vi "AlliGator Read metadata.txt File.vi"(8 "Error In":errorcluster, 11 "Folder Path":path) -> (0 "Error Out":errorcluster, 1 "Metadata":T1 {"Date" format="%<%x %.3X>T"}, 2 "AlliGator Version":string, 3 "Settings String":string)   [LabVIEW 2021, in "AlliGator Files.lvlib"]
doc: "Tries to extract FLI dataset metadata from a _metadata.txt file generated by AlliGator."
uses:
  AlliGator Files.lvlib
  AlliGator RecSettings Metadata.ctl
  AlliGator Gate Folder Metadata List.ctl
panel:
  # "see the AlliGator License on the block diagram (Ctrl+E or Window:Show Block Diagram)"
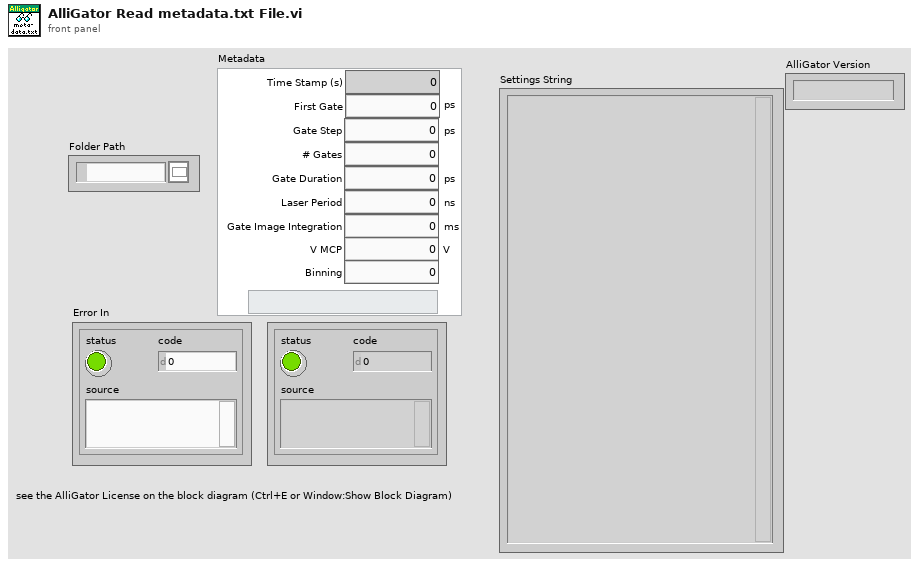
[diagram p1: front panel]
types:
  T1 = typedef "AlliGator Files.lvlib/AlliGator RecSettings Metadata.ctl" = cluster{"Time Stamp (s)":dbl, "First Gate":dbl[unit], "Gate Step":dbl[unit], "# Gates":i32, "Gate Duration":dbl[unit], "Laser Period":dbl[unit], "Gate Image Integration":dbl[unit], "Date":timestamp, "V MCP":dbl[unit], "Binning":dbl}
  T2 = typedef "AlliGator Files.lvlib/AlliGator Gate Folder Metadata List.ctl" = enum16{"[DAQ Parameters]", "DAQ Parameters.# Pixel X", "DAQ Parameters.# Pixel Y", "DAQ Parameters.# Gates", "DAQ Parameters.# Datasets", "DAQ Parameters.Exposure/Gate", "DAQ Parameters.Macrotime Gate Separation", "DAQ Parameters.Nanotime Gate Separation", "DAQ Parameters.Gate Duration", "DAQ Parameters.Laser Period", "[Dataset Timestamp]", "Timestamp", "[Metadata]", "AlliGator Version"}
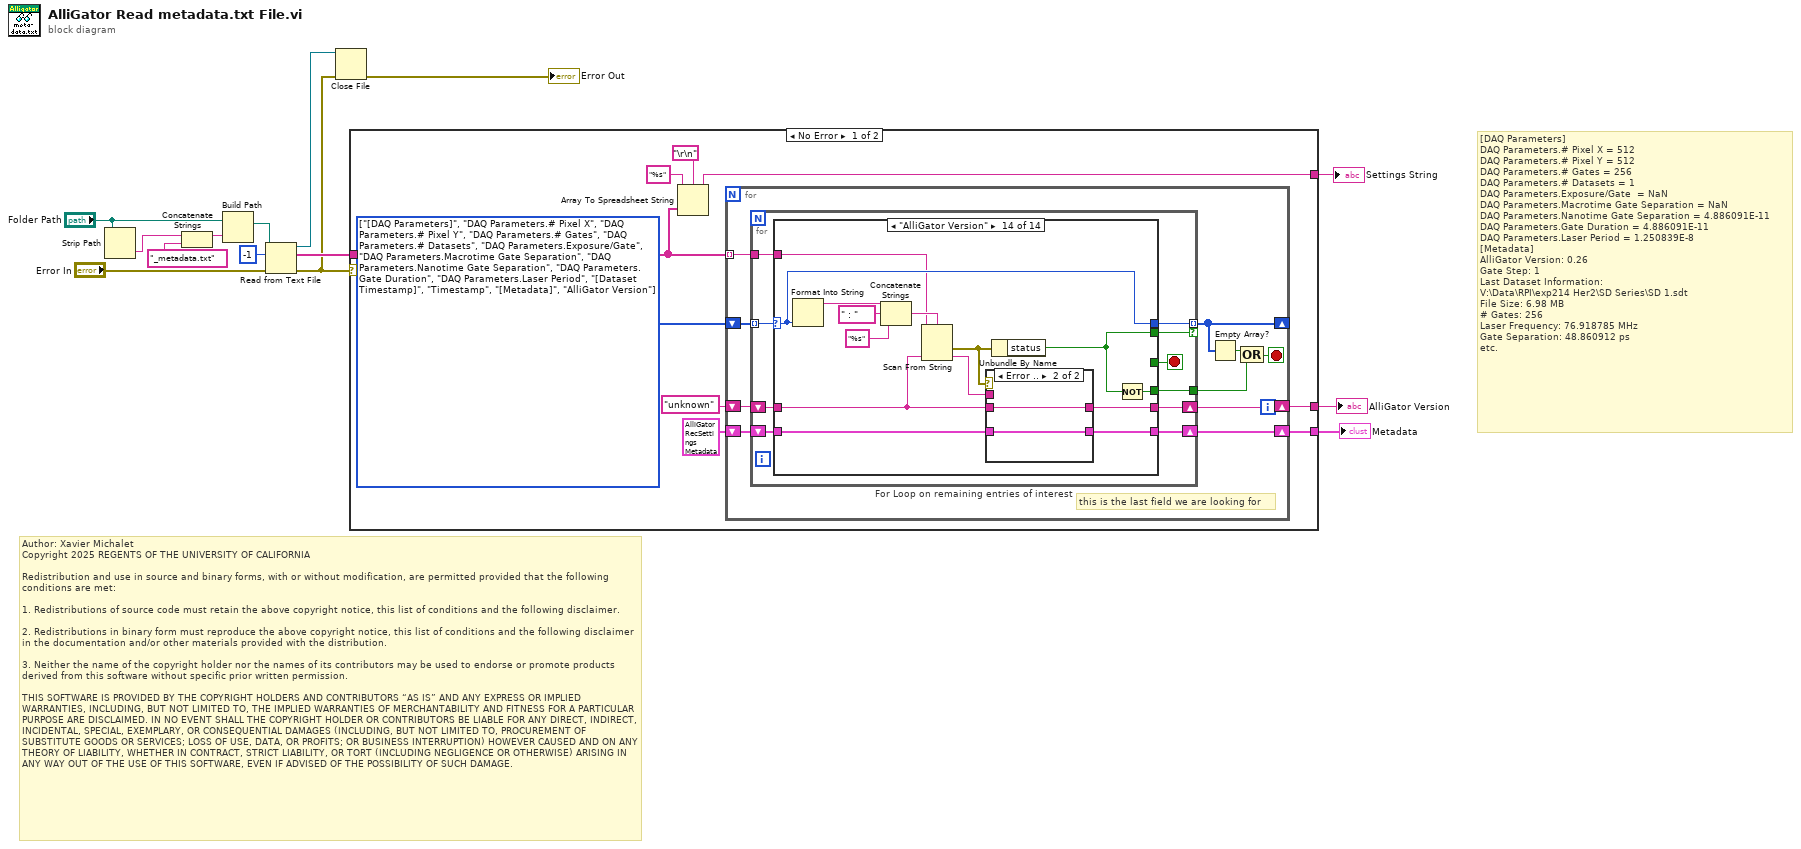
[diagram p0: block diagram]
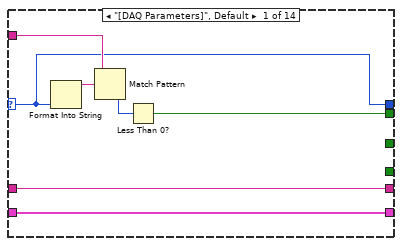
[diagram p2: hidden frame]
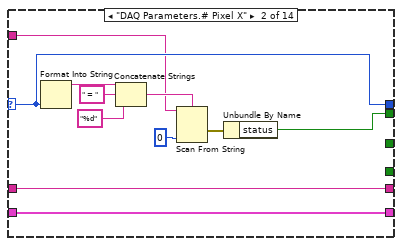
[diagram p3: hidden frame]
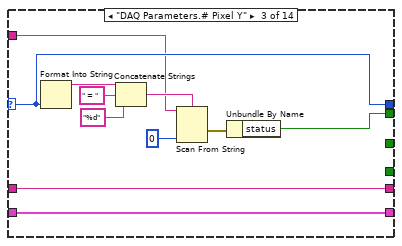
[diagram p4: hidden frame]
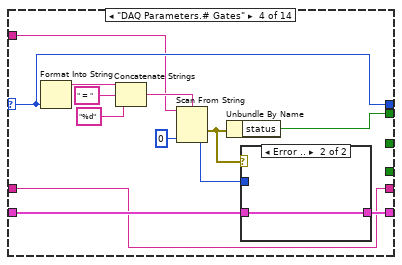
[diagram p5: hidden frame]
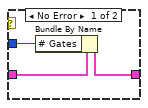
[diagram p6: hidden frame]
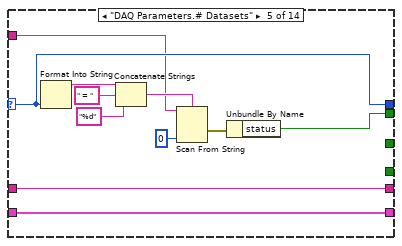
[diagram p7: hidden frame]
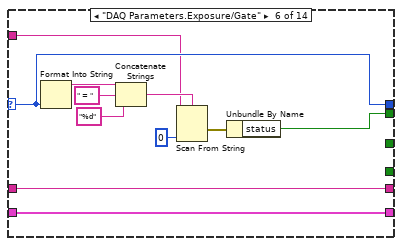
[diagram p8: hidden frame]
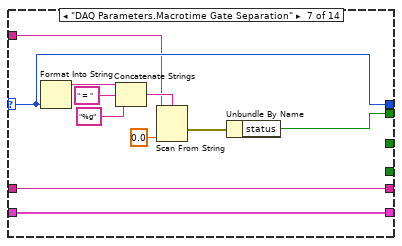
[diagram p9: hidden frame]
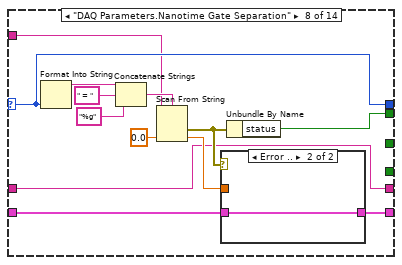
[diagram p10: hidden frame]
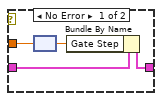
[diagram p11: hidden frame]
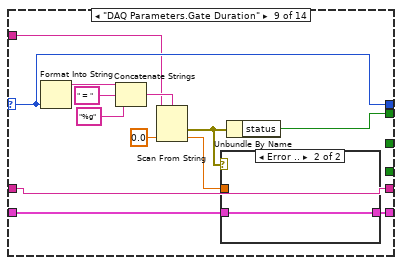
[diagram p12: hidden frame]
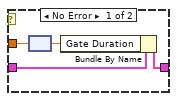
[diagram p13: hidden frame]
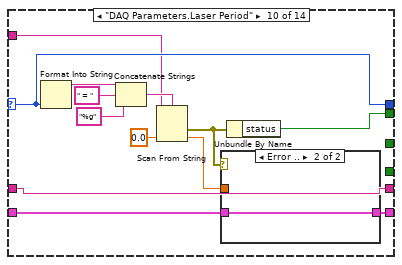
[diagram p14: hidden frame]
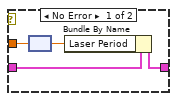
[diagram p15: hidden frame]
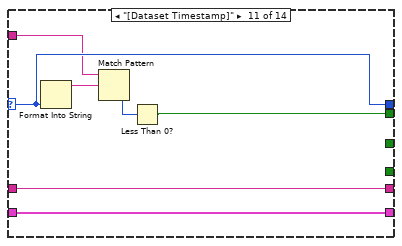
[diagram p16: hidden frame]
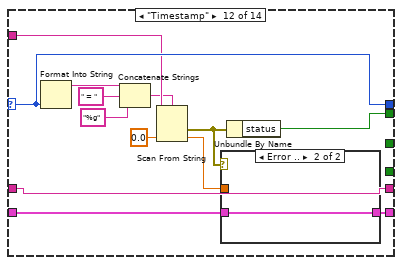
[diagram p17: hidden frame]
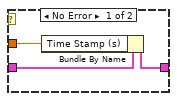
[diagram p18: hidden frame]
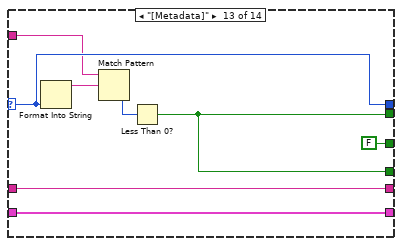
[diagram p19: hidden frame]
diagram:
  # "Author: Xavier Michalet\nCopyright 2025 REGENTS OF THE UNIVERSITY OF CALIFORNIA\n\nRedistribution and use in source and binary forms, with or without modification, are permitted provided that the following conditions are met:\n\n1. Redistributions of source code must retain the above copyright notice, this list of conditions and the following disclaimer.\n\n2. Redistributions in binary form must reproduce the above copyright notice, this list of conditions and the following disclaimer in the documentation and/or other materials provided with the distribution.\n\n3. Neither the name of the copyright holder nor the names of its contributors may be used to endorse or promote products derived from this software without specific prior written permission.\n\nTHIS SOFTWARE IS PROVIDED BY THE COPYRIGHT HOLDERS AND CONTRIBUTORS “AS IS” AND ANY EXPRESS OR IMPLIED WARRANTIES, INCLUDING, BUT NOT LIMITED TO, THE IMPLIED WARRANTIES OF MERCHANTABILITY AND FITNESS FOR A PARTICULAR PURPOSE ARE DISCLAIMED. IN NO EVENT SHALL THE COPYRIGHT HOLDER OR CONTRIBUTORS BE LIABLE FOR ANY DIRECT, INDIRECT, INCIDENTAL, SPECIAL, EXEMPLARY, OR CONSEQUENTIAL DAMAGES (INCLUDING, BUT NOT LIMITED TO, PROCUREMENT OF SUBSTITUTE GOODS OR SERVICES; LOSS OF USE, DATA, OR PROFITS; OR BUSINESS INTERRUPTION) HOWEVER CAUSED AND ON ANY THEORY OF LIABILITY, WHETHER IN CONTRACT, STRICT LIABILITY, OR TORT (INCLUDING NEGLIGENCE OR OTHERWISE) ARISING IN ANY WAY OUT OF THE USE OF THIS SOFTWARE, EVEN IF ADVISED OF THE POSSIBILITY OF SUCH DAMAGE."
  # "[DAQ Parameters]\nDAQ Parameters.# Pixel X = 512\nDAQ Parameters.# Pixel Y = 512\nDAQ Parameters.# Gates = 256\nDAQ Parameters.# Datasets = 1\nDAQ Parameters.Exposure/Gate  = NaN\nDAQ Parameters.Macrotime Gate Separation = NaN\nDAQ Parameters.Nanotime Gate Separation = 4.886091E-11\nDAQ Parameters.Gate Duration = 4.886091E-11\nDAQ Parameters.Laser Period = 1.250839E-8\n[Metadata]\nAlliGator Version: 0.26\nGate Step: 1\nLast Dataset Information:\nV:\\Data\\RPI\\exp214 Her2\\SD Series\\SD 1.sdt\nFile Size: 6.98 MB\n# Gates: 256\nLaser Frequency: 76.918785 MHz\nGate Separation: 48.860912 ps\netc."
  n1 = Strip Path(path="Folder Path") -> (name=w4:string)  [unwired: 1 out]
  n2 = Concatenate Strings(w4, "_metadata.txt" ("name or relative path")) -> (w2:string)
  n3 = Build Path(base path="Folder Path", name or relative path=w2) -> (appended path=w10:path)
  n4 = Read from Text File(file (use dialog)=w10, count=-1, error in="Error In") -> (refnum out=w14:refnum<file>, text=w13:string[], error out=w8:errorcluster)  [unwired: 1 in, 1 out]
  n5 = Close File(refnum=w14, error in=w8) -> (error out=→"Error Out":errorcluster)  [unwired: 1 out]
  n6 = case shown="No Error" w8 {
    tunnel: w13 -> [w20 _]
    tunnel: [w22 "No metadata  found..." ("spreadsheet string")] -> w12
    tunnel: [w18 _] -> w7
    tunnel: [w16 "unknown" ("string")] -> w1
    frame No Error {
      w19 = T2[] [enum."[DAQ Parameters]", enum."DAQ Parameters.# Pixel X", enum."DAQ Parameters.# Pixel Y", enum."DAQ Parameters.# Gates", enum."DAQ Parameters.# Datasets", enum."DAQ Parameters.Exposure/Gate", enum."DAQ Parameters.Macrotime Gate Separation", enum."DAQ Parameters.Nanotime Gate Separation", enum."DAQ Parameters.Gate Duration", enum."DAQ Parameters.Laser Period", enum."[Dataset Timestamp]", enum."Timestamp", enum."[Metadata]", enum."AlliGator Version"] items=["[DAQ Parameters]", "DAQ Parameters.# Pixel X", "DAQ Parameters.# Pixel Y", "DAQ Parameters.# Gates", "DAQ Parameters.# Datasets", "DAQ Parameters.Exposure/Gate", "DAQ Parameters.Macrotime Gate Separation", "DAQ Parameters.Nanotime Gate Separation", "DAQ Parameters.Gate Duration", "DAQ Parameters.Laser Period", "[Dataset Timestamp]", "Timestamp", "[Metadata]", "AlliGator Version"] ("Array")
      n7 = Array To Spreadsheet String(delimiter (Tab)="\r\n", array=w20, 3:"%s" ("format string")) -> (spreadsheet string=w22:string)
      n8 = for {
        shift-right: [w31] -> w18
        shift-left: T1 {"Time Stamp (s)"=nan, "First Gate"=nan, "Gate Step"=nan, "# Gates"=0, "Gate Duration"=nan, "Laser Period"=nan, "Gate Image Integration"=nan, "Date"=timestamp(0 s since 1904-01-01), "V MCP"=nan, "Binning"=nan} ("Metadata") -> [w32]
        tunnel: w20 -> [w30] mode=indexing
        shift-right: [w29] -> _
        shift-left: w19 -> [w33]
        shift-right: [w24] -> w16
        shift-left: "unknown" ("string") -> [w25]
        stop <- w27 stop-if-true
        # "this is the last field we are looking for"
        n9 = for "For Loop on remaining entries of interest" {
          tunnel: w33 -> [w43] mode=indexing
          shift-right: [w41] -> w31
          shift-left: w32 -> [w42]
          tunnel: w30 -> [w40]
          tunnel: [w39] -> w29 mode=indexing if=w37
          tunnel: [w36] -> w26
          shift-right: [w34] -> w24
          shift-left: w25 -> [w35]
          stop <- w38 stop-if-true
          n10 = case shown="\"AlliGator Version\"" w43 {
            selector: w43 -> [w47 w61 w72 w85 w100 w111 w122 w135 w153 w171 w183 w196 w208 w222]
            tunnel: w42 -> [w45 w60 w71 w77 w92 w103 w113 w126 w144 w162 w182 w191 w207 w215]
            tunnel: [w45 w60 w71 w76 w92 w103 w113 w125 w143 w161 w182 w190 w207 w214] -> w41
            tunnel: w40 -> [w49 w55 w66 w80 w95 w106 w117 w130 w148 w166 w179 w195 w204 w217]
            tunnel: [w47 w61 w72 w85 w100 w111 w122 w135 w153 w171 w183 w196 w208 w222] -> w39
            tunnel: [w48 w52 w63 w78 w93 w104 w115 w128 w146 w164 w178 w193 w203 w210] -> w37
            tunnel: [_ _ _ _ _ _ _ _ _ _ _ _ FALSE _] -> w38
            tunnel: [_ _ _ _ _ _ _ _ _ _ _ _ w203 w209] -> w36
            tunnel: w35 -> [w44 w51 w62 w73 w90 w101 w112 w123 w141 w159 w177 w184 w201 w211]
            tunnel: [w44 w51 w62 w73 w90 w101 w112 w123 w141 w159 w177 w184 w201 w212] -> w34
            frame "[DAQ Parameters]", Default {
              n11 = Format Into String(w47) -> (resulting string=w46:string)  [unwired: 3 in, 1 out]
              n12 = Match Pattern(string=w49, regular expression=w46) -> (offset past match=w50:i32)  [unwired: 1 in, 3 out]
              n13 = Less Than 0?(x=w50) -> (x < 0?=w48:bool)
            }
            frame "DAQ Parameters.# Pixel X" {
              n14 = Format Into String(w61) -> (resulting string=w59:string)  [unwired: 3 in, 1 out]
              n15 = Concatenate Strings(w59, " = " ("string"), "%d" ("string")) -> (w56:string)
              n16 = Scan From String(format string=w56, input string=w55, default 1=0 ("default value 1")) -> (error out=w53:errorcluster)  [unwired: 3 in, 2 out]
              n17 = Unbundle By Name(w53) -> ("status"=w52:bool)
            }
            frame "DAQ Parameters.# Pixel Y" {
              n18 = Format Into String(w72) -> (resulting string=w70:string)  [unwired: 3 in, 1 out]
              n19 = Concatenate Strings(w70, " = " ("string"), "%d" ("string")) -> (w67:string)
              n20 = Scan From String(format string=w67, input string=w66, default 1=0 ("default value 1")) -> (error out=w64:errorcluster)  [unwired: 3 in, 2 out]
              n21 = Unbundle By Name(w64) -> ("status"=w63:bool)
            }
            frame "DAQ Parameters.# Gates" {
              n22 = Format Into String(w85) -> (resulting string=w84:string)  [unwired: 3 in, 1 out]
              n23 = Concatenate Strings(w84, " = " ("string"), "%d" ("string")) -> (w81:string)
              n24 = Scan From String(format string=w81, input string=w80, default 1=0 ("default value 1")) -> (error out=w75:errorcluster, output 1=w74:i32)  [unwired: 2 in, 2 out]
              n25 = Unbundle By Name(w75) -> ("status"=w78:bool)
              n26 = case shown="Error .." w75 {
                tunnel: w77 -> [w88 w89]
                tunnel: [w87 w89] -> w76
                tunnel: w74 -> [w86 _]
                frame No Error {
                  n27 = Bundle By Name(cluster=w88, "# Gates"=w86) -> (w87:T1)
                }
                frame Error {
                }
              }
            }
            frame "DAQ Parameters.# Datasets" {
              n28 = Format Into String(w100) -> (resulting string=w99:string)  [unwired: 3 in, 1 out]
              n29 = Concatenate Strings(w99, " = " ("string"), "%d" ("string")) -> (w96:string)
              n30 = Scan From String(format string=w96, input string=w95, default 1=0 ("default value 1")) -> (error out=w91:errorcluster)  [unwired: 3 in, 2 out]
              n31 = Unbundle By Name(w91) -> ("status"=w93:bool)
            }
            frame "DAQ Parameters.Exposure/Gate" {
              n32 = Format Into String(w111) -> (resulting string=w110:string)  [unwired: 3 in, 1 out]
              n33 = Concatenate Strings(w110, " = " ("string"), "%d" ("string")) -> (w107:string)
              n34 = Scan From String(format string=w107, input string=w106, default 1=0 ("default value 1")) -> (error out=w102:errorcluster)  [unwired: 3 in, 2 out]
              n35 = Unbundle By Name(w102) -> ("status"=w104:bool)
            }
            frame "DAQ Parameters.Macrotime Gate Separation" {
              n36 = Format Into String(w122) -> (resulting string=w121:string)  [unwired: 3 in, 1 out]
              n37 = Concatenate Strings(w121, " = " ("string"), "%g" ("string")) -> (w118:string)
              n38 = Scan From String(format string=w118, input string=w117, default 1=0.0 ("default value 1")) -> (error out=w114:errorcluster)  [unwired: 3 in, 2 out]
              n39 = Unbundle By Name(w114) -> ("status"=w115:bool)
            }
            frame "DAQ Parameters.Nanotime Gate Separation" {
              n40 = Format Into String(w135) -> (resulting string=w134:string)  [unwired: 3 in, 1 out]
              n41 = Concatenate Strings(w134, " = " ("string"), "%g" ("string")) -> (w131:string)
              n42 = Scan From String(format string=w131, input string=w130, default 1=0.0 ("default value 1")) -> (error out=w127:errorcluster, output 1=w124:dbl)  [unwired: 2 in, 2 out]
              n43 = case shown="Error .." w127 {
                tunnel: w126 -> [w139 w140]
                tunnel: [w138 w140] -> w125
                tunnel: w124 -> [w137 _]
                frame No Error {
                  n44 = node(w137) -> (w136:dbl[unit])
                  n45 = Bundle By Name(cluster=w139, "Gate Step"=w136) -> (w138:T1)
                }
                frame Error {
                }
              }
              n46 = Unbundle By Name(w127) -> ("status"=w128:bool)
            }
            frame "DAQ Parameters.Gate Duration" {
              n47 = Format Into String(w153) -> (resulting string=w152:string)  [unwired: 3 in, 1 out]
              n48 = Concatenate Strings(w152, " = " ("string"), "%g" ("string")) -> (w149:string)
              n49 = Scan From String(format string=w149, input string=w148, default 1=0.0 ("default value 1")) -> (error out=w145:errorcluster, output 1=w142:dbl)  [unwired: 2 in, 2 out]
              n50 = case shown="Error .." w145 {
                tunnel: w144 -> [w157 w158]
                tunnel: [w156 w158] -> w143
                tunnel: w142 -> [w155 _]
                frame No Error {
                  n51 = node(w155) -> (w154:dbl[unit])
                  n52 = Bundle By Name(cluster=w157, "Gate Duration"=w154) -> (w156:T1)
                }
                frame Error {
                }
              }
              n53 = Unbundle By Name(w145) -> ("status"=w146:bool)
            }
            frame "DAQ Parameters.Laser Period" {
              n54 = Format Into String(w171) -> (resulting string=w170:string)  [unwired: 3 in, 1 out]
              n55 = Concatenate Strings(w170, " = " ("string"), "%g" ("string")) -> (w167:string)
              n56 = Scan From String(format string=w167, input string=w166, default 1=0.0 ("default value 1")) -> (error out=w163:errorcluster, output 1=w160:dbl)  [unwired: 2 in, 2 out]
              n57 = case shown="Error .." w163 {
                tunnel: w162 -> [w175 w176]
                tunnel: [w174 w176] -> w161
                tunnel: w160 -> [w173 _]
                frame No Error {
                  n58 = node(w173) -> (w172:dbl[unit])
                  n59 = Bundle By Name(cluster=w175, "Laser Period"=w172) -> (w174:T1)
                }
                frame Error {
                }
              }
              n60 = Unbundle By Name(w163) -> ("status"=w164:bool)
            }
            frame "[Dataset Timestamp]" {
              n61 = Format Into String(w183) -> (resulting string=w180:string)  [unwired: 3 in, 1 out]
              n62 = Match Pattern(string=w179, regular expression=w180) -> (offset past match=w181:i32)  [unwired: 1 in, 3 out]
              n63 = Less Than 0?(x=w181) -> (x < 0?=w178:bool)
            }
            frame "Timestamp" {
              n64 = Format Into String(w196) -> (resulting string=w186:string)  [unwired: 3 in, 1 out]
              n65 = Concatenate Strings(w186, " = " ("string"), "%g" ("string")) -> (w185:string)
              n66 = Scan From String(format string=w185, input string=w195, default 1=0.0 ("default value 1")) -> (error out=w192:errorcluster, output 1=w189:dbl)  [unwired: 2 in, 2 out]
              n67 = case shown="Error .." w192 {
                tunnel: w191 -> [w199 w200]
                tunnel: [w198 w200] -> w190
                tunnel: w189 -> [w197 _]
                frame No Error {
                  n68 = Bundle By Name(cluster=w199, "Time Stamp (s)"=w197) -> (w198:T1)
                }
                frame Error {
                }
              }
              n69 = Unbundle By Name(w192) -> ("status"=w193:bool)
            }
            frame "[Metadata]" {
              n70 = Format Into String(w208) -> (resulting string=w205:string)  [unwired: 3 in, 1 out]
              n71 = Match Pattern(string=w204, regular expression=w205) -> (offset past match=w206:i32)  [unwired: 1 in, 3 out]
              n72 = Less Than 0?(x=w206) -> (x < 0?=w203:bool)
            }
            frame "AlliGator Version" {
              n73 = Format Into String(w222) -> (resulting string=w221:string)  [unwired: 3 in, 1 out]
              n74 = Concatenate Strings(w221, " : " ("string"), "%s" ("string")) -> (w218:string)
              n75 = Scan From String(format string=w218, input string=w217, default 1=w211) -> (error out=w216:errorcluster, output 1=w213:string)  [unwired: 2 in, 2 out]
              n76 = case shown="Error .." w216 {
                tunnel: w215 -> [w224 w226]
                tunnel: [w224 w226] -> w214
                tunnel: w213 -> [w223 _]
                tunnel: [w223 w225] -> w212
                tunnel: w211 -> [_ w225]
                frame No Error {
                }
                frame Error {
                }
              }
              n77 = Unbundle By Name(w216) -> ("status"=w210:bool)
              n78 = Not(x=w210) -> (.not. x?=w209:bool)
            }
          }
        }
        n79 = Empty Array?(array=w29) -> (empty?=w28:bool)
        n80 = Compound Arithmetic op=OR(w28, w26) -> (w27:bool)
      }
    }
    frame Error {
    }
  }
  "Settings String" <- w12
  "Metadata" <- w7
  "AlliGator Version" <- w1
